vi "myRIO_BRig SPI MISO.vi"(7 "Index":T1, 8 "Sample?":bool, 9 "LSB first?":bool, 10 "MISO":bool, 11 "Reset?":bool) -> (3 "Data In":u16)   [LabVIEW 2014]
uses:
  myRIO_BRig SPI Frame Length.ctl
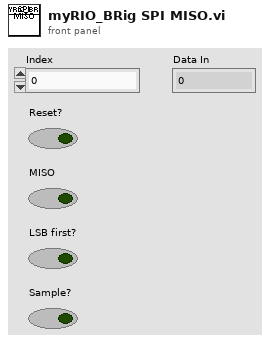
[diagram p1: front panel]
types:
  T1 = typedef "myRIO_BRig SPI Frame Length.ctl" = fxp<+,4,4>
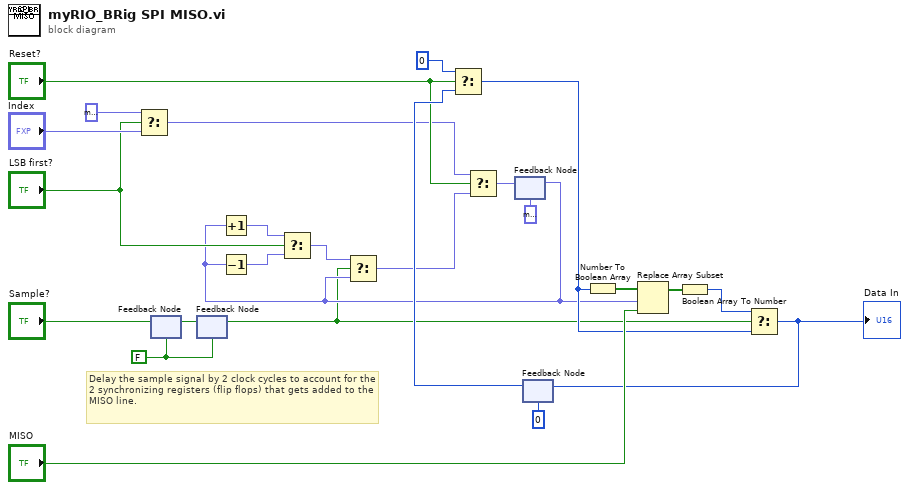
[diagram p0: block diagram]
diagram:
  w1 = FALSE ("Sample?")
  # "Delay the sample signal by 2 clock cycles to account for the 2 synchronizing registers (flip flops) that gets added to the MISO line."
  n1 = Select(t=T1 0.0, s="LSB first?", f="Index") -> (s? t:f=w14:T1)
  n2 = feedback-in #1("Sample?") -> ()
  n3 = feedback #1(w1) -> (w3:bool)
  n4 = feedback-in #2(w3) -> ()
  n5 = feedback #2(w1) -> (w2:bool)
  n6 = feedback #3(T1 0.0 ("Index")) -> (w4:T1)
  n7 = Increment(x=w4) -> (x+1=w11:T1)
  n8 = Decrement(x=w4) -> (x-1=w10:T1)
  n9 = Select(t=w11, s="LSB first?", f=w10) -> (s? t:f=w9:T1)
  n10 = Select(t=w9, s=w2, f=w4) -> (s? t:f=w8:T1)
  n11 = Select(t=w14, s="Reset?", f=w8) -> (s? t:f=w13:T1)
  n12 = feedback-in #3(w13) -> ()
  n13 = feedback #4(u16 0 ("Data In")) -> (w19:u16)
  n14 = Select(t=u16 0 ("Data In"), s="Reset?", f=w19) -> (s? t:f=w16:u16)
  n15 = Number To Boolean Array(number=w16) -> (Boolean array=w24:bool[])
  n16 = Replace Array Subset(array=w24, new element="MISO", index=w4) -> (w23:bool[])
  n17 = Boolean Array To Number(Boolean array=w23) -> (number=w17:u16)
  n18 = Select(t=w17, s=w2, f=w16) -> (s? t:f=w20:u16)
  "Data In" <- w20
  n19 = feedback-in #4(w20) -> ()
